vi "Vesta_Reconnect_Check.vi"(8 "error in":errorcluster, 9 "Vesta Is Working":bool) -> (0 "error out":errorcluster, 2 "Display Data?":bool, 3 "Count":dbl)   [LabVIEW 2020]
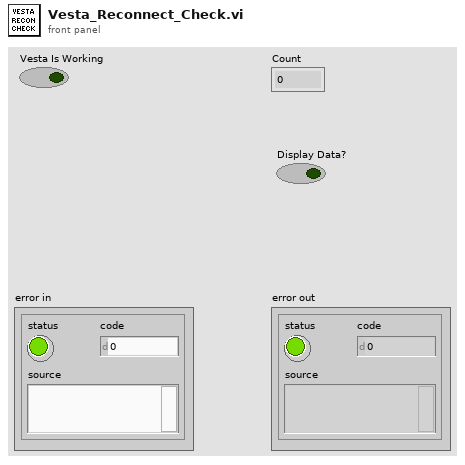
[diagram p1: front panel]
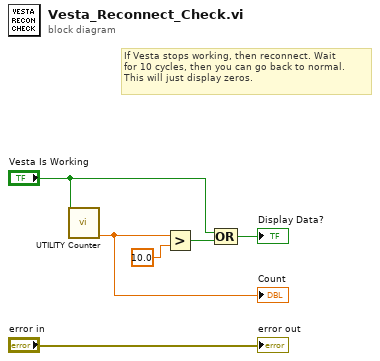
[diagram p0: block diagram]
diagram:
  # "If Vesta stops working, then reconnect. Wait\nfor 10 cycles, then you can go back to normal. \nThis will just display zeros."
  n1 = call "UTILITY Counter.vi"("Reset"="Vesta Is Working") -> ("Count"=w5:dbl)  [unwired: 10 in]
  "Count" <- w5
  n2 = Greater?(x=w5, y=10.0) -> (0:w3:bool)
  n3 = Compound Arithmetic op=OR("Vesta Is Working", w3) -> (→"Display Data?":bool)
  "error out" <- "error in"
